vi "Measure_Valve.vi"(8 "error in (no error)":errorcluster, 10 "Parameters":string, 11 "reference in":refnum<class "Test_Flux_Capacitor.lvclass">) -> (0 "error out":errorcluster, 2 "Result":dbl, 3 "reference out":refnum<class "Test_Flux_Capacitor.lvclass">)   [LabVIEW 2022 SP3, in "Test_Flux_Capacitor.lvlib" / "Test_Flux_Capacitor.lvclass"]
uses:
  Test_Flux_Capacitor.lvclass
  ParameterTypes/MeasureValve.ctl
  ParameterTypes/DMM_DCV.vi
  Components/SwitchBase.lvlibp/SwitchBase.lvclass
  Components/DMM_Keysight_34980A.lvlibp/DMM_Keysight_34980A.lvclass
  <vilib>/JDP Science/JSONtext/JSONtext.lvlib
panel:
  in  "Parameter_Type":T1={"Pre_Switch"="", "Post_Switch"="", "Wait (msec)"=0, "Scale"=0.0, "DMM_DCV"={"Range "=enum."Auto", "Resolution"=enum."Default", "Samples"=1, "dt (s)"=0.0, "Timeout (s)"=10000.0}, "Valve_State"=FALSE, "Valve"=enum."1"}
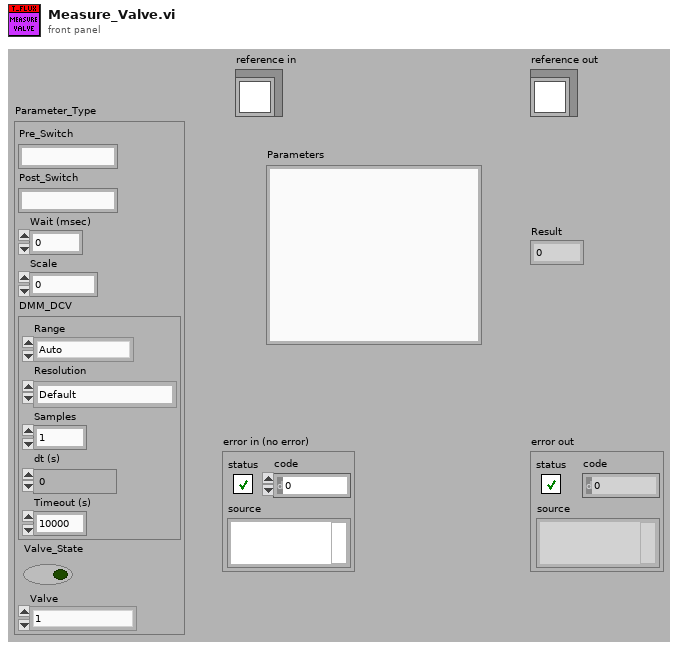
[diagram p1: front panel]
types:
  T1 = typedef "Test_Flux_Capacitor.lvlib/Test_Flux_Capacitor.lvclass/MeasureValve.ctl" = cluster{"Pre_Switch":string, "Post_Switch":string, "Wait (msec)":u32, "Scale":dbl, "DMM_DCV":T2, "Valve_State":bool, "Valve":enum16{"1", "2", "3", "4", "5", "6", "7", "8", "v_drain", "v_small", "v_large", "v_pump", "v_temp"}}
  T2 = typedef "Test_Flux_Capacitor.lvlib/Test_Flux_Capacitor.lvclass/DMM_DCV.vi" = cluster{"Range ":enum16{"100 mV", "1 V", "10 V", "100 V", "300 V", "Auto", "Minimum", "Maximum"}, "Resolution":enum16{"4 1/2", "5 1/2", "6 1/2", "Least", "Highest", "Default"}, "Samples":u32, "dt (s)":dbl, "Timeout (s)":dbl}
  T3 = typedef "Test_Flux_Capacitor.lvlib/Test_Flux_Capacitor.lvclass/ObjectAttributes.ctl" = cluster{"Config":T4, "DMM":refnum<class "DMM_Keysight_34980A.lvclass">, "LCR":refnum<class "LCR_BK891.lvclass">, "PSU":refnum<class "PSU_Base.lvclass">, "Switch_Manager":refnum<class "SwitchBase.lvclass">, "FRAM":string, "Flux_Capacitor":refnum<class "Flux_Capacitor.lvclass">, "Frequency_Counter":refnum<class "Frequency_Counter_Base.lvclass">, "JTAG":refnum<class "JTAG_Base.lvclass">}
  T4 = typedef "Test_Flux_Capacitor.lvlib/Test_Flux_Capacitor.lvclass/Config.ctl" = cluster{"default":string}
  T5 = enum16{"100 mV", "1 V", "10 V", "100 V", "300 V", "Auto", "Minimum", "Maximum"}
  T6 = enum16{"4 1/2", "5 1/2", "6 1/2", "Least", "Highest", "Default"}
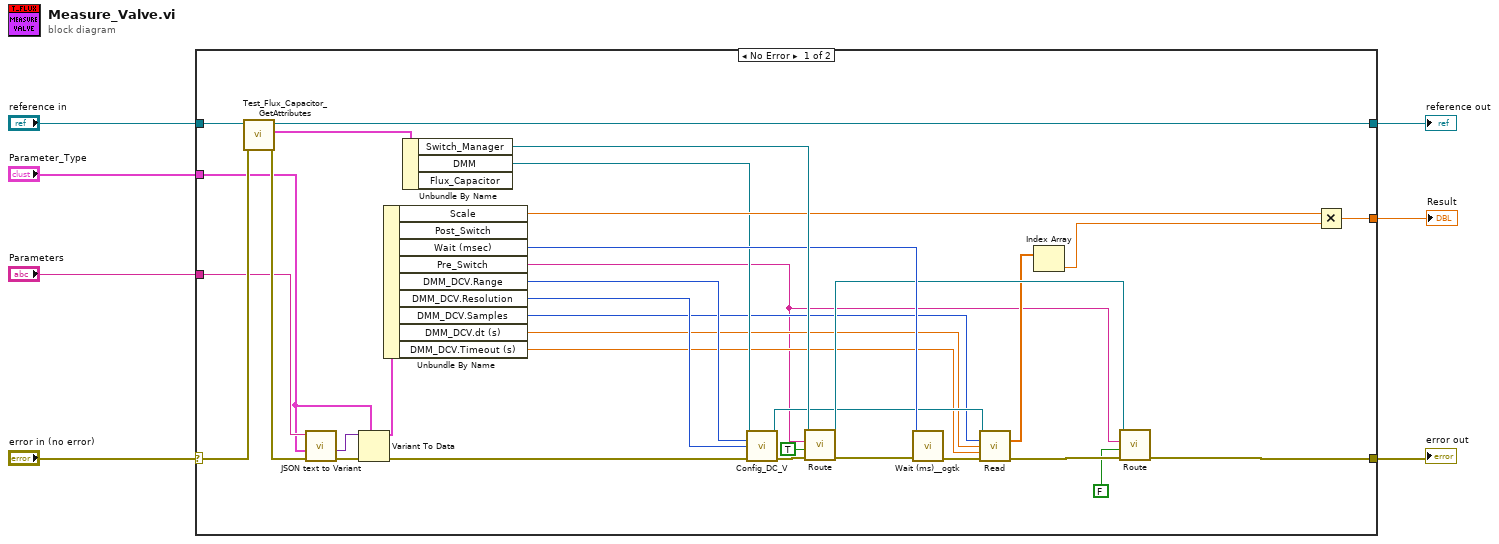
[diagram p0: block diagram]
diagram:
  n1 = case shown="No Error" "error in (no error)" {
    selector: "error in (no error)" -> [w40 w42]
    tunnel: [w20 w42] -> w6
    tunnel: [w38 w41] -> w4
    tunnel: "reference in" -> [w39 w41]
    tunnel: "Parameters" -> [w14 _]
    tunnel: "Parameter_Type" -> [w9 _]
    tunnel: [w31 _] -> w1
    frame No Error {
      n2 = call "Test_Flux_Capacitor_GetAttributes.vi"("error in (no error)"=w40, "reference in"=w39) -> ("error out"=w16:errorcluster, "Data"=w37:T3, "reference out"=w38:refnum<class "Test_Flux_Capacitor.lvclass">)  [unwired: 6 in, 1 out]
      n3 = call <vilib>:"JSON text to Variant.vi"("error in (no error)"=w16, "Data Type"=w9, "JSON"=w14) -> ("error out"=w15:errorcluster, "Variant out"=w13:variant)  [unwired: 7 in]
      n4 = Variant To Data(error in=w15, type=w9, Variant=w13) -> (data=w36:T1, error out=w21:errorcluster)
      n5 = Unbundle By Name(w36) -> ("Scale"=w32:dbl, "Wait (msec)"=w34:u32, "Pre_Switch"=w12:string, "DMM_DCV.Range"=w26:T5, "DMM_DCV.Resolution"=w25:T6, "DMM_DCV.Samples"=w19:u32, "DMM_DCV.dt (s)"=w18:dbl, "DMM_DCV.Timeout (s)"=w17:dbl)  [unwired: 1 out]
      n6 = Unbundle By Name(w37) -> ("Switch_Manager"=w35:refnum<class "SwitchBase.lvclass">, "DMM"=w24:refnum<class "DMM_Keysight_34980A.lvclass">)  [unwired: 1 out]
      n7 = call-dynamic "Config_DC_V.vi"("reference in"=w24, "Range (5:Auto)"=w26, "Resolution (5:Default)"=w25, "error in (no error)"=w21) -> ("reference in"=w22:refnum<class "DMM_Keysight_34980A.lvclass">, "error out"=w23:errorcluster)  [unwired: 10 in]
      n8 = call-dynamic "Route.vi"("error in (no error)"=w23, "Connect"=TRUE, "channel 1"=w12, "reference in"=w35) -> ("error out"=w8:errorcluster, "reference in"=w33:refnum<class "SwitchBase.lvclass">)  [unwired: 6 in]
      n9 = call <userlib>:"Wait (ms)__ogtk.vi"("error in (no error)"=w8, "milliseconds to wait"=w34) -> ("error out"=w30:errorcluster)  [unwired: 8 in, 1 out]
      n10 = call-dynamic "Read.vi"("reference in"=w22, "Samples"=w19, "dt"=w18, "Timeout (10 s)"=w17, "error in (no error)"=w30) -> ("Measurement"=w28:dbl[], "error out"=w29:errorcluster)  [unwired: 7 in, 2 out]
      n11 = Index Array(array=w28) -> (element=w27:dbl)  [unwired: 1 in]
      n12 = call-dynamic "Route.vi"("error in (no error)"=w29, "Connect"=FALSE, "channel 1"=w12, "reference in"=w33) -> ("error out"=w20:errorcluster)  [unwired: 6 in, 1 out]
      n13 = Multiply(x=w32, y=w27) -> (x*y=w31:dbl)
    }
    frame Error {
    }
  }
  "Result" <- w1
  "error out" <- w6
  "reference out" <- w4
